vi "ToMatlabNamePath.vi"(11 "MatlabDataBundle":T1) -> (3 "NamePath":string[](array[string]))   [LabVIEW 2017]
uses:
  Types/MatlabDataBundle.ctl
  Types/MatlabDataType.ctl
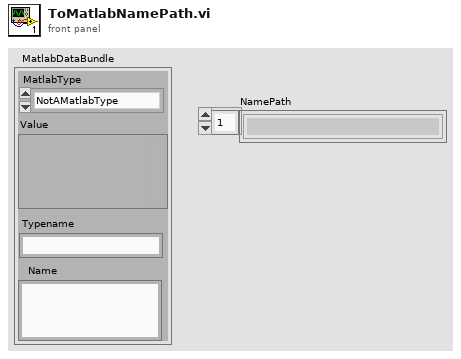
[diagram p1: front panel]
types:
  T1 = typedef "MatlabDataBundle.ctl" = cluster{"MatlabType":T2, "Value":variant, "Name":string, "Typename":string}
  T2 = typedef "MatlabDataType.ctl" = enum16{"NotAMatlabType", "Real", "Complex", "String", "Boolean"}
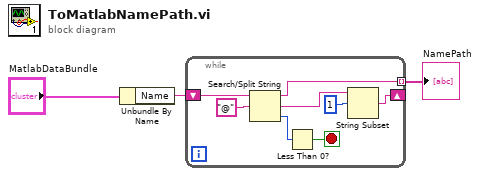
[diagram p0: block diagram]
diagram:
  n1 = Unbundle By Name("MatlabDataBundle") -> ("Name"=w1:string)
  n2 = while {
    tunnel: [w10] -> w2 mode=indexing
    shift-right: [w4] -> _
    shift-left: w1 -> [w7]
    stop <- w8 stop-if-true
    n3 = Search/Split String(string=w7, search string/char (-)="@") -> (substring before match=w10:string, match + rest of string=w5:string, offset of match=w9:i32)  [unwired: 1 in]
    n4 = Less Than 0?(x=w9) -> (x < 0?=w8:bool)
    n5 = String Subset(string=w5, offset (0)=1) -> (substring=w4:string)  [unwired: 1 in]
  }
  "NamePath" <- w2
